vi "Initialize ReadWrite Data.vi"(8 "error in (no error)":errorcluster, 10 "Chan Refs":T1[](array[typedef]) format="%.0x", 11 "Name":string) -> (0 "error out":errorcluster, 3 "ReadWrite Data":T2 {"Pairs"."Chan Refs" format="%.0x"})   [LabVIEW 2015, in "Diagnostics Addon Engine.lvlib" / "Inline Async API.lvlib"]
uses:
  Inline Async API.lvlib
  Controls/ReadWrite Data.ctl
  <vilib>/NI Veristand/Custom Device API/Data Reference.ctl
  <vilib>/NI Veristand/Custom Device API/Custom Device API.lvlib
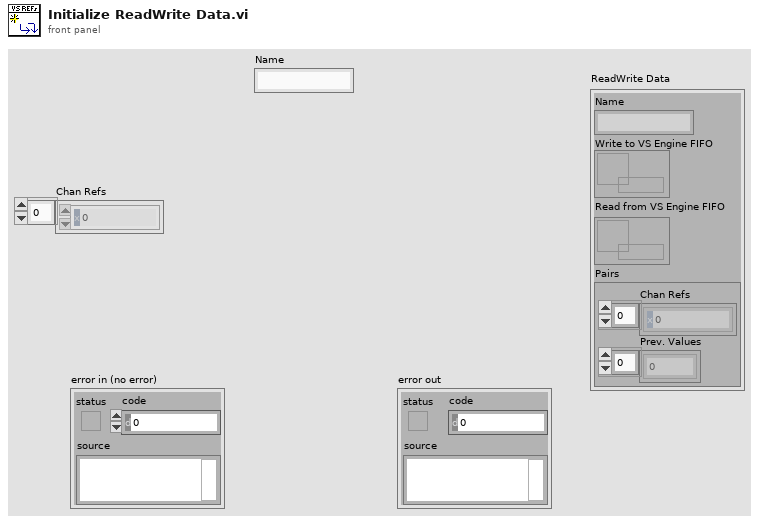
[diagram p1: front panel]
types:
  T1 = typedef "Custom Device API.lvlib/Data Reference.ctl" = i32
  T2 = typedef "Diagnostics Addon Engine.lvlib/Inline Async API.lvlib/ReadWrite Data.ctl" = cluster{"Name":string, "Write to VS Engine FIFO":refnum<k33>, "Read from VS Engine FIFO":refnum<k33>, "Pairs":cluster{"Chan Refs":T1[], "Prev. Values":dbl[]}}
  T3 = cluster{"read mode":enum16{"polling", "blocking"}, "write mode":enum16{"polling", "blocking"}}
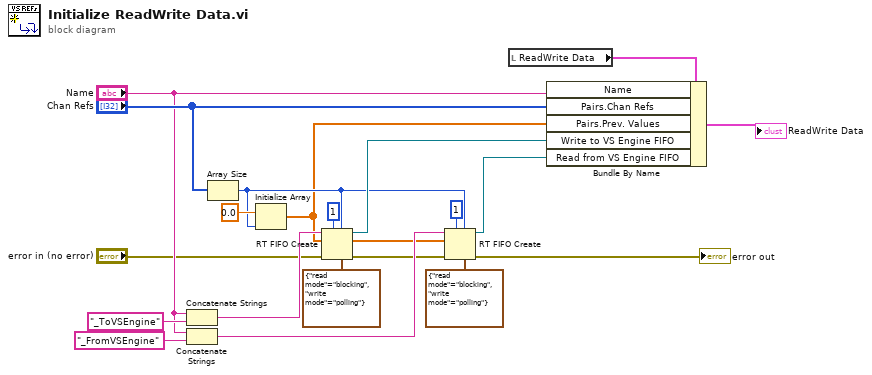
[diagram p0: block diagram]
diagram:
  n1 = Concatenate Strings("Name", "_ToVSEngine" ("string")) -> (w10:string)
  n2 = Concatenate Strings("Name", "_FromVSEngine" ("string")) -> (w9:string)
  n3 = Array Size(array="Chan Refs") -> (size(s)=w7:i32)
  n4 = Initialize Array(0.0 ("element"), w7) -> (w6:dbl[])
  n5 = RT FIFO Create(0:w10, 1:w6, 3:"error in (no error)", 4:u32 1 ("size (10)"), 6:w7, 7:T3 {"read mode"=enum."blocking", "write mode"=enum."polling"} ("r/w modes (polling,polling)")) -> (8:w18:refnum<k33>, 11:w5:errorcluster)  [unwired: 2 in, 1 out]
  n6 = RT FIFO Create(0:w9, 1:w6, 3:w5, 4:u32 1 ("size (10)"), 6:w7, 7:T3 {"read mode"=enum."blocking", "write mode"=enum."polling"} ("r/w modes (polling,polling)")) -> (8:w19:refnum<k33>, 11:→"error out":errorcluster)  [unwired: 2 in, 1 out]
  n7 = local read "ReadWrite Data"() -> (w4:T2)
  n8 = Bundle By Name(cluster=w4, "Name"="Name", "Pairs.Chan Refs"="Chan Refs", "Pairs.Prev. Values"=w6, "Write to VS Engine FIFO"=w18, "Read from VS Engine FIFO"=w19) -> (→"ReadWrite Data":T2)
